vi "Host Main.vi"() -> ()   [LabVIEW 2019]
uses:
  <userlib>/_NI SPI IP/FPGA/Controllers/Public/Transfer Settings.ctl
  <vilib>/FPGAPlugInAG/sbRIO-9651/niLvFpga_Open_sbRIO-9651.vi
  <vilib>/Utility/error.llb/Error Cluster From Error Code.vi
  <vilib>/rvi/errors/niLvFpgaAdjustHostInterfaceError.vi
  <vilib>/FPGAPlugInAG/sbRIO-9651/niLvFpga_Run_sbRIO-9651.vi
  <vilib>/FPGAPlugInAG/sbRIO-9651/niLvFpga_Abort_sbRIO-9651.vi
  <vilib>/FPGAPlugInAG/sbRIO-9651/niLvFpga_Close_sbRIO-9651.vi
  <vilib>/rvi/interface/nirviOpenFPGA/nirviOpenFPGA.xnode
  FPGA Bitfiles/adafruitlcdsom_FPGATarget_FPGAMain_K7l+4zj6vFY.lvbitx
  FPGA Main.vi
  <vilib>/rvi/interface/nirviReadWriteControl/nirviReadWriteControl.xnode
  <vilib>/rvi/interface/nirviMethod/nirviMethod.xnode
  TypeDefs/FPGA Reference.ctl
  <vilib>/rvi/interface/nirviCloseFPGA/nirviCloseFPGA.xnode
  <vilib>/rvi/errors/niLvFpgaMergeErrorWithErrorCode.vi
  <userlib>/_NI SPI IP/FPGA/Controllers/NI SPI IP FPGA.lvlib
  <vilib>/FPGAPlugInAG/sbRIO-9651/niLvFpga_StartFifo_sbRIO-9651.vi
  NiFpgaLv.dll
panel:
  in  "Master Settings":T1={"Divide Value"=1, "Transfer Length (bits)"=8, "CS Asserted Polarity"=FALSE, "Clock Polarity (CPOL)"=FALSE, "Clock Phase (CPHA)"=FALSE, "Lengthen MISO Setup"=FALSE, "Direction Change Bit"=0, "MOSI Starts as Output"=FALSE, "Tristatable MOSI"=FALSE} {"Direction Change Bit" max=64 step=1; "Transfer Length (bits)" min=1 max=64 step=1}
  out "error out":errorcluster
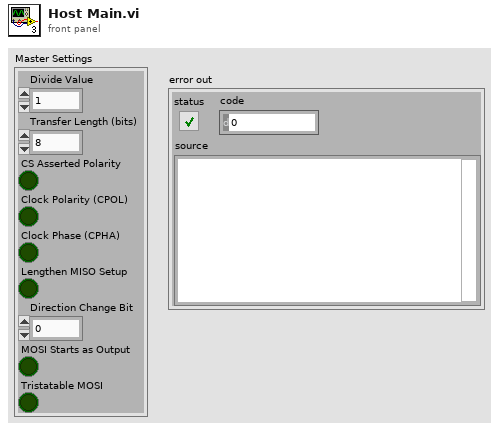
[diagram p1: front panel]
types:
  T1 = typedef "NI SPI IP FPGA.lvlib/Transfer Settings.ctl" = cluster{"Divide Value":u8, "Transfer Length (bits)":u8, "CS Asserted Polarity":bool, "Clock Polarity (CPOL)":bool, "Clock Phase (CPHA)":bool, "Lengthen MISO Setup":bool, "Direction Change Bit":u8, "MOSI Starts as Output":bool, "Tristatable MOSI":bool}
  T2 = typedef "FPGA Reference.ctl" = refnum<k20>
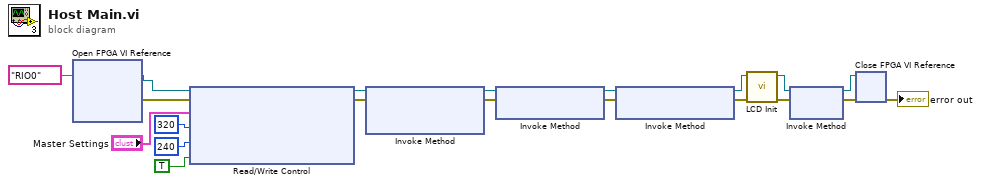
[diagram p0: block diagram]
diagram:
  n1 = xnode "Open FPGA VI Reference"("resource name"=tag "RIO0") -> ("FPGA VI Reference Out"=w1:refnum<k20>, "error out"=w20:errorcluster)  [unwired: 1 in]
  n2 = xnode "Read/Write Control"("FPGA VI Reference In"=w1, "error in"=w20, "Master Settings"="Master Settings", "Width"=320, "Height"=240, "StreamDisabled"=TRUE) -> ("FPGA VI Reference Out"=w5:refnum<k20>, "error out"=w4:errorcluster)
  n3 = xnode "Invoke Method"("FPGA VI Reference In"=w5, "error in"=w4) -> ("FPGA VI Reference Out"=w2:refnum<k20>, "error out"=w3:errorcluster)  [unwired: 1 in]
  n4 = xnode "Invoke Method"("FPGA VI Reference In"=w2, "error in"=w3) -> ("FPGA VI Reference Out"=w13:refnum<k20>, "error out"=w12:errorcluster)
  n5 = xnode "Invoke Method"("FPGA VI Reference In"=w13, "error in"=w12) -> ("FPGA VI Reference Out"=w11:refnum<k20>, "error out"=w10:errorcluster)
  n6 = call "LCD Init.vi"("error in"=w10, "FPGA VI Reference in"=w11) -> ("error out"=w16:errorcluster, "FPGA VI Reference Out"=w17:T2)  [unwired: 8 in]
  n7 = xnode "Invoke Method"("FPGA VI Reference In"=w17, "error in"=w16) -> ("FPGA VI Reference Out"=w14:T2, "error out"=w15:errorcluster)
  n8 = xnode "Close FPGA VI Reference"("FPGA VI Reference In"=w14, "error in"=w15) -> ("error out"=→"error out":errorcluster)
